vi "Wave1D_Init Data_BC.vi"(9 "delta x":dbl, 10 "ks":dbl, 11 "Boundary Condition":cluster{"type":T1, "Value":dbl[]}[](array[cluster]) {"type" items=["Dirichlet", "Neumann"]}) -> (3 "BC":T2 {"End X"."type" items=["Dirichlet", "Neumann"]; "Start X"."type" items=["Dirichlet", "Neumann"]})   [LabVIEW 2017, in "NI_PDE.lvlib"]
uses:
  <vilib>/gmath/NI_PDE.lvlib
  <vilib>/gmath/pde.llb/Common/PDE_BC Type.ctl
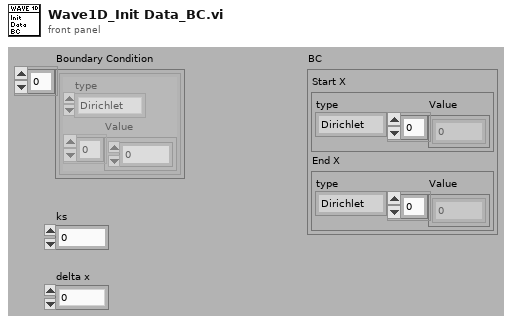
[diagram p1: front panel]
types:
  T1 = typedef "NI_PDE.lvlib/PDE_BC Type.ctl" = i32
  T2 = cluster{"Start X":cluster{"type":T1, "Value":dbl[]}, "End X":cluster{"type":T1, "Value":dbl[]}}
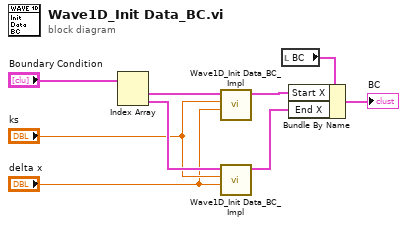
[diagram p0: block diagram]
diagram:
  n1 = Index Array(array="Boundary Condition") -> (element #1=w8:cluster{"type":T1, "Value":dbl[]}, element #2=w7:cluster{"type":T1, "Value":dbl[]})  [unwired: 2 in]
  n2 = call <vilib>:"Wave1D_Init Data_BC_Impl.vi"("delta x"="delta x", "ks"="ks", "Boundary Condition"=w8) -> ("BC"=w3:cluster{"type":T1, "Value":dbl[]})  [unwired: 8 out]
  n3 = call <vilib>:"Wave1D_Init Data_BC_Impl.vi"("delta x"="delta x", "ks"="ks", "Boundary Condition"=w7) -> ("BC"=w2:cluster{"type":T1, "Value":dbl[]})  [unwired: 8 out]
  n4 = local read "BC"() -> (w4:T2)
  n5 = Bundle By Name(cluster=w4, "Start X"=w3, "End X"=w2) -> (→"BC":T2)
